vi "Get Terminals.vi"(8 "error in (no error)":errorcluster, 11 "Reference":refnum<vi>) -> (0 "error out":errorcluster, 1 "Array of terminals":refnum<vi>[](array[refnum]), 3 "First Terminal":refnum<vi>)   [LabVIEW 2012, in "Scripting Tools.lvlib"]
doc: "Gets the terminal references from various GObject references. Returns the first terminal and an array of all terminals (for object which only have one terminal, the array contains just the single terminal."
uses:
  <userlib>/_LAVAcr/Scripting Tools/Scripting Tools.lvlib
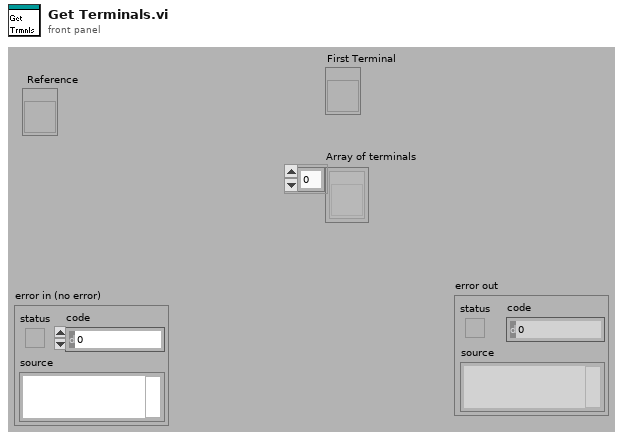
[diagram p1: front panel]
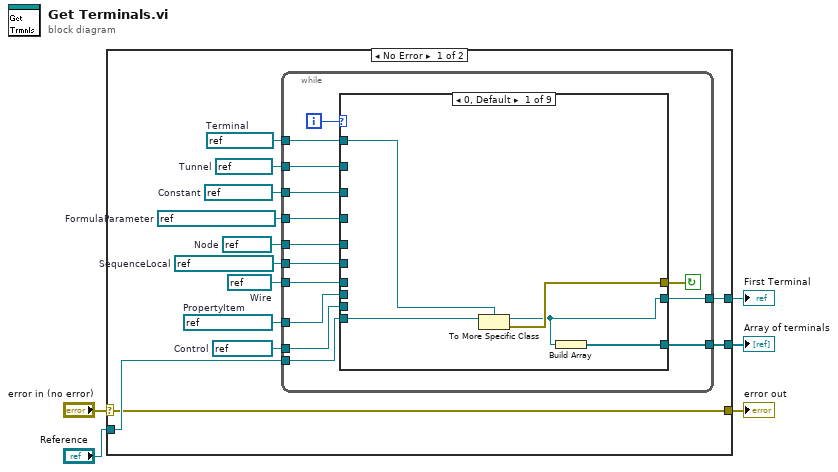
[diagram p0: block diagram]
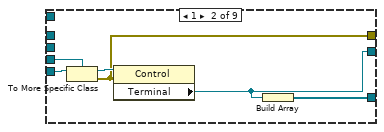
[diagram p2: hidden frame]
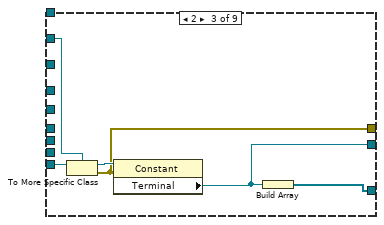
[diagram p3: hidden frame]
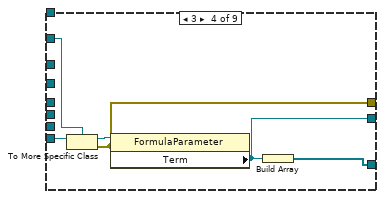
[diagram p4: hidden frame]
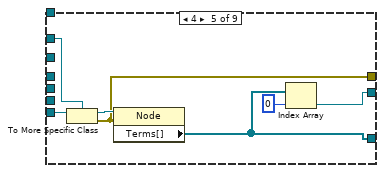
[diagram p5: hidden frame]
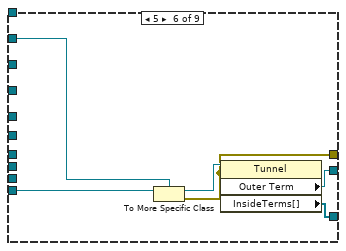
[diagram p6: hidden frame]
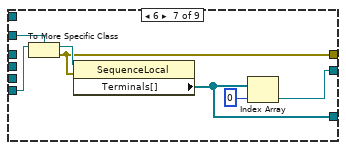
[diagram p7: hidden frame]
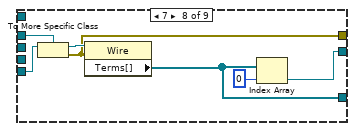
[diagram p8: hidden frame]
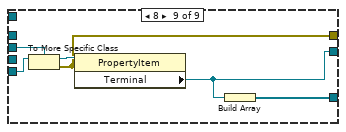
[diagram p9: hidden frame]
diagram:
  n1 = case shown="No Error" "error in (no error)" {
    selector: "error in (no error)" -> [w6 w89]
    tunnel: "Reference" -> [w18 _]
    tunnel: [w15 _] -> w4
    tunnel: [w10 _] -> w3
    tunnel: [w6 w89] -> w1
    frame No Error {
      w7 = refnum<vi> refnum  # PropertyItem
      w8 = refnum<vi> refnum  # Wire
      w9 = refnum<vi> refnum  # SequenceLocal
      w11 = refnum<vi> refnum  # Tunnel
      w12 = refnum<vi> refnum  # Node
      w13 = refnum<vi> refnum  # FormulaParameter
      w14 = refnum<vi> refnum  # Constant
      w16 = refnum<vi> refnum  # Control
      w17 = refnum<vi> refnum  # Terminal
      n2 = while {
        tunnel: w18 -> [w32]
        tunnel: w17 -> [w30]
        tunnel: [w28] -> w15
        tunnel: w16 -> [w27]
        tunnel: w14 -> [w26]
        tunnel: w13 -> [w25]
        tunnel: w12 -> [w24]
        tunnel: w11 -> [w23]
        tunnel: [w22] -> w10
        tunnel: w9 -> [w21]
        tunnel: w8 -> [w20]
        tunnel: w7 -> [w19]
        i -> [w31]
        stop <- w29 continue-if-true
        n3 = case shown="0, Default" w31 {
          tunnel: w32 -> [w37 w43 w49 w55 w62 w68 w75 w82 w88]
          tunnel: w30 -> [w36 _ _ _ _ _ _ _ _]
          tunnel: [w35 w38 w44 w50 w56 w63 w69 w76 w83] -> w29
          tunnel: [w34 w40 w46 w52 w59 w65 w73 w80 w84] -> w28
          tunnel: w27 -> [_ w42 _ _ _ _ _ _ _]
          tunnel: w26 -> [_ _ w47 _ _ _ _ _ _]
          tunnel: w25 -> [_ _ _ w53 _ _ _ _ _]
          tunnel: w24 -> [_ _ _ _ w60 _ _ _ _]
          tunnel: w23 -> [_ _ _ _ _ w66 _ _ _]
          tunnel: [w33 w39 w45 w51 w57 w64 w70 w77 w86] -> w22
          tunnel: w21 -> [_ _ _ _ _ _ w71 _ _]
          tunnel: w20 -> [_ _ _ _ _ _ _ w78 _]
          tunnel: w19 -> [_ _ _ _ _ _ _ _ w85]
          frame 0, Default {
            n4 = To More Specific Class(target class=w36, reference=w37) -> (specific class reference=w34:refnum<vi>, error out=w35:errorcluster)  [unwired: 1 in]
            n5 = Build Array(w34) -> (w33:refnum<vi>[])
          }
          frame 1 {
            n6 = To More Specific Class(target class=w42, reference=w43) -> (specific class reference=w41:refnum<vi>, error out=w38:errorcluster)  [unwired: 1 in]
            n7 = property on="Property Node" class="Control"(reference=w41, error in=w38) -> ("Terminal"=w40:refnum<vi>)  [unwired: 2 out]
            n8 = Build Array(w40) -> (w39:refnum<vi>[])
          }
          frame 2 {
            n9 = To More Specific Class(target class=w47, reference=w49) -> (specific class reference=w48:refnum<vi>, error out=w44:errorcluster)  [unwired: 1 in]
            n10 = property on="Property Node" class="Constant"(reference=w48, error in=w44) -> ("Terminal"=w46:refnum<vi>)  [unwired: 2 out]
            n11 = Build Array(w46) -> (w45:refnum<vi>[])
          }
          frame 3 {
            n12 = To More Specific Class(target class=w53, reference=w55) -> (specific class reference=w54:refnum<vi>, error out=w50:errorcluster)  [unwired: 1 in]
            n13 = property on="Property Node" class="FormulaParameter"(reference=w54, error in=w50) -> ("Term"=w52:refnum<vi>)  [unwired: 2 out]
            n14 = Build Array(w52) -> (w51:refnum<vi>[])
          }
          frame 4 {
            n15 = To More Specific Class(target class=w60, reference=w62) -> (specific class reference=w61:refnum<vi>, error out=w56:errorcluster)  [unwired: 1 in]
            n16 = property on="Property Node" class="Node"(reference=w61, error in=w56) -> ("Terms[]"=w57:refnum<vi>[])  [unwired: 2 out]
            n17 = Index Array(array=w57, index=0) -> (element=w59:refnum<vi>)
          }
          frame 5 {
            n18 = To More Specific Class(target class=w66, reference=w68) -> (specific class reference=w67:refnum<vi>, error out=w63:errorcluster)  [unwired: 1 in]
            n19 = property on="Property Node" class="Tunnel"(reference=w67, error in=w63) -> ("Outer Term"=w65:refnum<vi>, "InsideTerms[]"=w64:refnum<vi>[])  [unwired: 2 out]
          }
          frame 6 {
            n20 = To More Specific Class(target class=w71, reference=w75) -> (specific class reference=w74:refnum<vi>, error out=w69:errorcluster)  [unwired: 1 in]
            n21 = property on="Property Node" class="SequenceLocal"(reference=w74, error in=w69) -> ("Terminals[]"=w70:refnum<vi>[])  [unwired: 2 out]
            n22 = Index Array(array=w70, index=0) -> (element=w73:refnum<vi>)
          }
          frame 7 {
            n23 = To More Specific Class(target class=w78, reference=w82) -> (specific class reference=w81:refnum<vi>, error out=w76:errorcluster)  [unwired: 1 in]
            n24 = property on="Property Node" class="Wire"(reference=w81, error in=w76) -> ("Terms[]"=w77:refnum<vi>[])  [unwired: 2 out]
            n25 = Index Array(array=w77, index=0) -> (element=w80:refnum<vi>)
          }
          frame 8 {
            n26 = To More Specific Class(target class=w85, reference=w88) -> (specific class reference=w87:refnum<vi>, error out=w83:errorcluster)  [unwired: 1 in]
            n27 = property on="Property Node" class="PropertyItem"(reference=w87, error in=w83) -> ("Terminal"=w84:refnum<vi>)  [unwired: 2 out]
            n28 = Build Array(w84) -> (w86:refnum<vi>[])
          }
        }
      }
    }
    frame Error {
    }
  }
  "First Terminal" <- w4
  "Array of terminals" <- w3
  "error out" <- w1
